vi "PID_OL_AM.vi"(5 "reinitialize? (F)":bool, 6 "manual control":dbl format="%.2f", 7 "X1(SetState)":T1(ring)=enum."max", 8 "dt (s) in":dbl=-1.0, 9 "process variable":dbl step=0.01 format="%.2f", 10 "setpoint":dbl step=0.01 format="%.2f", 11 "PID in":refnum<class "PID_OL_AM.lvclass">) -> (0 "dt out (s)":dbl format="%.3f", 1 "rate lim output":dbl format="%.2f", 2 "pid output":dbl format="%.2f", 3 "PID out":refnum<class "PID_OL_AM.lvclass">)   [LabVIEW 2019, in "control.lvlib" / "PID_OL_AM.lvclass"]
uses:
  PID_OL_AM.lvclass
  D:/my_projects/projects/Algorithms/Labview/19/Reg/PID/PID Timing Estimation/PID Timing Estimation.lvclass
  D:/my_projects/projects/Algorithms/Labview/19/Reg/PID/PID Output Rate Limiter/PID Output Rate Limiter.lvclass
  PID Timing Estimation/PID Timing Estimation.lvclass/PID Timing Estimation.ctl
  PID Output Rate Limiter/PID Output Rate Limiter.lvclass/PID Output Rate Limiter.ctl
  PID_OL_AM.lvclass/PID_OL_AM.ctl
  PID Output Rate Limiter/PID Output Rate Limiter.lvclass
  PID Timing Estimation/PID Timing Estimation.lvclass
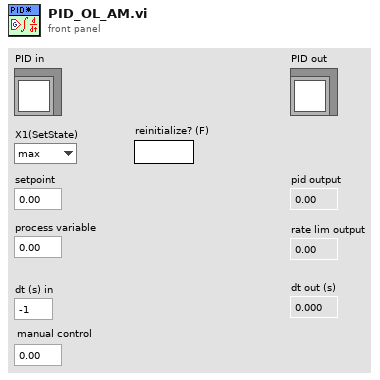
[diagram p1: front panel]
types:
  T1 = enum8{"alarm", "min", "stop", "hand", "auto", "max"}
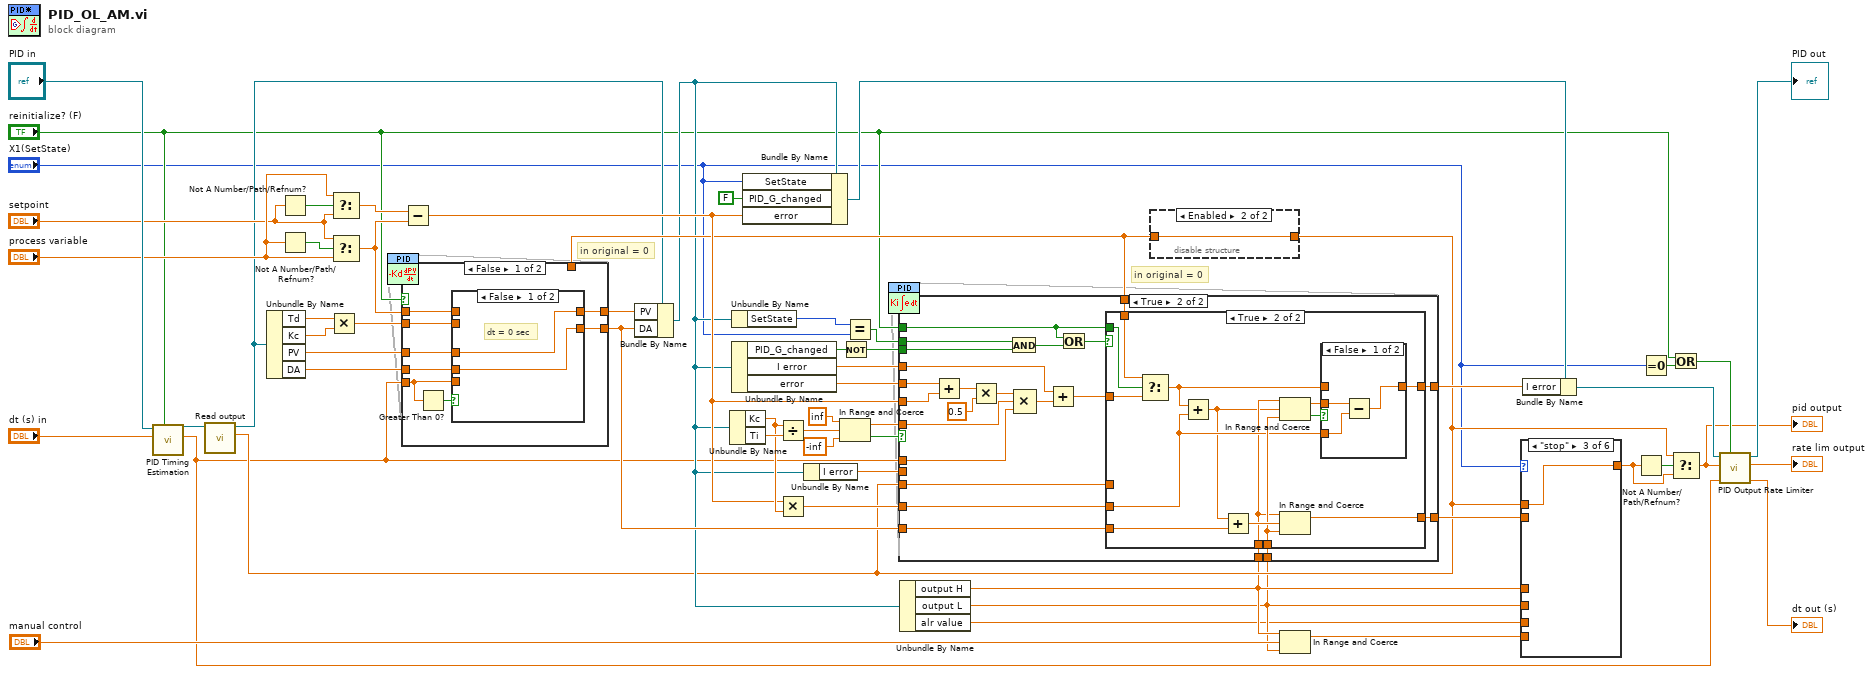
[diagram p0: block diagram]
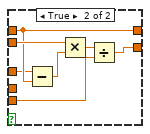
[diagram p7: hidden frame]
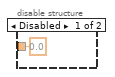
[diagram p9: hidden frame]
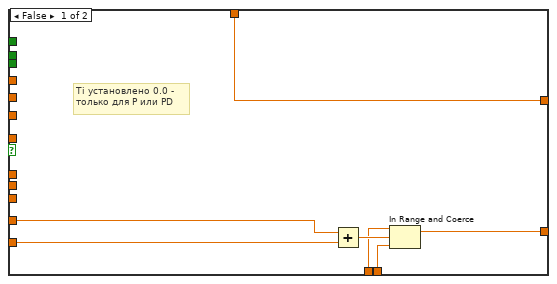
[diagram p10: hidden frame]
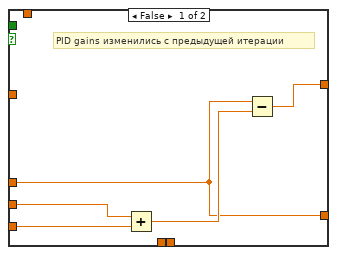
[diagram p11: hidden frame]
diagram:
  # "in original = 0"
  # "in original = 0"
  n1 = call "PID Timing Estimation.vi"("R"="reinitialize? (F)", "dt (s) in"="dt (s) in", "PID Timing Estimation in"="PID in") -> ("dt (s) out"=w4:dbl, "PID Timing Estimation out"=w26:refnum<class "PID_OL_AM.lvclass">)  [unwired: 7 in]
  n2 = call "Read output.vi"("PID Output Rate Limiter in"=w26) -> ("output"=w8:dbl, "PID Output Rate Limiter out"=w25:refnum<class "PID_OL_AM.lvclass">)  [unwired: 9 in]
  n3 = Unbundle By Name(w25) -> ("Td"=w41:dbl, "Kc"=w44:dbl, "PV"=w43:dbl, "DA"=w40:dbl)
  n4 = Not A Number/Path/Refnum?(number/path/refnum="setpoint") -> (NaN/Path/Refnum?=w48:bool)
  n5 = Not A Number/Path/Refnum?(number/path/refnum="process variable") -> (NaN/Path/Refnum?=w49:bool)
  n6 = Multiply(x=w41, y=w44) -> (x*y=w52:dbl)
  n7 = Select(t="process variable", s=w48, f="setpoint") -> (s? t:f=w47:dbl)
  n8 = Select(t="setpoint", s=w49, f="process variable") -> (s? t:f=w30:dbl)
  n9 = Subtract(x=w47, y=w30) -> (x-y=w31:dbl)
  n10 = disable-structure shown="Enabled" {
    disable-tunnel: [0.0 ("output") w59] -> w29
    disable-tunnel: w8 -> [_ w59]
    frame Disabled {
    }
    frame Enabled {
    }
  }
  n11 = case shown="False" "reinitialize? (F)" {
    tunnel: w43 -> [w67 _]
    tunnel: w52 -> [w64 _]
    tunnel: w30 -> [w66 w78]
    tunnel: [w63 w78] -> w37
    tunnel: [w65 w77] -> w36
    tunnel: w40 -> [w61 _]
    tunnel: w4 -> [w60 _]
    tunnel: w29 -> [_ w77]
    frame False {
      n12 = Greater Than 0?(x=w60) -> (x > 0?=w62:bool)
      n13 = case shown="False" w62 {
        tunnel: w67 -> [w69 w70]
        tunnel: w60 -> [_ w75]
        tunnel: w66 -> [_ w71]
        tunnel: [w68 w74] -> w65
        tunnel: w64 -> [_ w73]
        tunnel: [w69 w71] -> w63
        tunnel: w61 -> [w68 _]
        frame False {
          # "dt = 0 sec"
        }
        frame True {
          n14 = Subtract(x=w70, y=w71) -> (x-y=w72:dbl)
          n15 = Multiply(x=w73, y=w72) -> (x*y=w76:dbl)
          n16 = Divide(x=w76, y=w75) -> (x/y=w74:dbl)
        }
      }
    }
    frame True {
    }
  }
  n17 = Bundle By Name(cluster=w25, "PV"=w37, "DA"=w36) -> (w14:refnum<class "PID_OL_AM.lvclass">)
  n18 = Unbundle By Name(w14) -> ("Kc"=w35:dbl, "Ti"=w42:dbl)
  n19 = Unbundle By Name(w14) -> ("SetState"=w13:T1)
  n20 = Unbundle By Name(w14) -> ("PID_G_changed"=w34:bool, "I error"=w33:dbl, "error"=w39:dbl)
  n21 = Bundle By Name(cluster=w14, "SetState"="X1(SetState)", "PID_G_changed"=FALSE, "error"=w31) -> (w18:refnum<class "PID_OL_AM.lvclass">)
  n22 = Divide(x=w35, y=w42) -> (x/y=w51:dbl)
  n23 = Multiply(x=w31, y=w35) -> (x*y=w50:dbl)
  n24 = Unbundle By Name(w14) -> ("I error"=w38:dbl)
  n25 = In Range and Coerce(upper limit=inf, x=w51, lower limit=-inf) -> (coerced(x)=w54:dbl, In Range?=w53:bool)
  n26 = Not(x=w34) -> (.not. x?=w2:bool)
  n27 = Equal?(x=w13, y="X1(SetState)") -> (x = y?=w12:bool)
  n28 = Unbundle By Name(w14) -> ("output H"=w7:dbl, "output L"=w6:dbl, "alr value"=w3:dbl)
  n29 = case shown="True" w53 {
    tunnel: w39 -> [_ w107]
    tunnel: w31 -> [_ w108]
    tunnel: w38 -> [_ _]
    tunnel: [w79 w100] -> w28
    tunnel: w54 -> [_ w98]
    tunnel: w50 -> [w84 w103]
    tunnel: [w85 w99] -> w22
    tunnel: w8 -> [_ w101]
    tunnel: w36 -> [w83 w97]
    tunnel: "reinitialize? (F)" -> [_ w96]
    tunnel: w2 -> [_ w86]
    tunnel: w4 -> [_ w95]
    tunnel: w7 -> [w81 w93]
    tunnel: w6 -> [w80 w94]
    tunnel: w29 -> [w79 w92]
    tunnel: w33 -> [_ w89]
    tunnel: w12 -> [_ w87]
    frame False {
      # "Ti установлено 0.0 -\nтолько для P или PD"
      n30 = Add(x=w84, y=w83) -> (x+y=w82:dbl)
      n31 = In Range and Coerce(upper limit=w81, x=w82, lower limit=w80) -> (coerced(x)=w85:dbl)  [unwired: 1 out]
    }
    frame True {
      n32 = Add(x=w107, y=w108) -> (x+y=w106:dbl)
      n33 = Multiply(x=w106, y=0.5) -> (x*y=w105:dbl)
      n34 = And(x=w87, y=w86) -> (x .and. y?=w88:bool)
      n35 = Compound Arithmetic op=MULTIPLY(w105, w98, w95) -> (w90:dbl)
      n36 = Add(x=w89, y=w90) -> (x+y=w104:dbl)
      n37 = Or(x=w96, y=w88) -> (x .or. y?=w102:bool)
      n38 = case shown="True" w102 {
        tunnel: w104 -> [_ w114]
        tunnel: w103 -> [w112 w120]
        tunnel: w101 -> [w109 _]
        tunnel: w96 -> [_ w117]
        tunnel: [w113 w122] -> w100
        tunnel: [w109 w126] -> w99
        tunnel: w97 -> [w111 w125]
        tunnel: w94 -> [_ w124]
        tunnel: w93 -> [_ w119]
        tunnel: w92 -> [_ w116]
        frame False {
          # "PID gains изменились с предыдущей итерации"
          n39 = Add(x=w112, y=w111) -> (x+y=w110:dbl)
          n40 = Subtract(x=w109, y=w110) -> (x-y=w113:dbl)
        }
        frame True {
          n41 = Select(t=w116, s=w117, f=w114) -> (s? t:f=w115:dbl)
          n42 = Add(x=w115, y=w120) -> (x+y=w118:dbl)
          n43 = Add(x=w118, y=w125) -> (x+y=w127:dbl)
          n44 = In Range and Coerce(upper limit=w119, x=w118, lower limit=w124) -> (coerced(x)=w121:dbl, In Range?=w123:bool)
          n45 = In Range and Coerce(upper limit=w119, x=w127, lower limit=w124) -> (coerced(x)=w126:dbl)  [unwired: 1 out]
          n46 = case shown="False" w123 {
            tunnel: w115 -> [_ w131]
            tunnel: [w128 w131] -> w122
            tunnel: w121 -> [w130 _]
            tunnel: w120 -> [w129 _]
            frame False {
              n47 = Subtract(x=w130, y=w129) -> (x-y=w128:dbl)
            }
            frame True {
            }
          }
        }
      }
    }
  }
  n48 = In Range and Coerce(upper limit=w7, x="manual control", lower limit=w6) -> (coerced(x)=w9:dbl)  [unwired: 1 out]
  n49 = case shown="\"stop\"" "X1(SetState)" {
    tunnel: w8 -> [_ _ w134 _ _ _]
    tunnel: w22 -> [_ _ _ _ w136 _]
    tunnel: w9 -> [_ _ _ w135 _ _]
    tunnel: [w132 w133 w134 w135 w136 w137] -> w23
    tunnel: w3 -> [w132 _ _ _ _ _]
    tunnel: w7 -> [_ _ _ _ _ w137]
    tunnel: w6 -> [_ w133 _ _ _ _]
    frame "alarm", Default {
    }
    frame "min" {
    }
    frame "stop" {
    }
    frame "hand" {
    }
    frame "auto" {
    }
    frame "max" {
    }
  }
  n50 = Bundle By Name(cluster=w18, "I error"=w28) -> (w17:refnum<class "PID_OL_AM.lvclass">)
  n51 = Not A Number/Path/Refnum?(number/path/refnum=w23) -> (NaN/Path/Refnum?=w24:bool)
  n52 = Equal To 0?(x="X1(SetState)") -> (x = 0?=w11:bool)
  n53 = Or(x="reinitialize? (F)", y=w11) -> (x .or. y?=w20:bool)
  n54 = Select(t=w8, s=w24, f=w23) -> (s? t:f=w1:dbl)
  "pid output" <- w1
  n55 = call "PID Output Rate Limiter.vi"("reinitialize? (F)"=w20, "dt (s)"=w4, "input (controller output)"=w1, "PID Output Rate Limiter in"=w17) -> ("dt (s) out"=→"dt out (s)":dbl, "output"=→"rate lim output":dbl, "PID Output Rate Limiter out"=→"PID out":refnum<class "PID_OL_AM.lvclass">)  [unwired: 5 in]
